vi "UserVars-Expand Repeat Value.vi"(7 "Expression":string) -> (8 "repeated values":dbl[](array[numeric]))   [LabVIEW 2020]
uses:
  <vilib>/regexp/Match Regular Expression.xnode
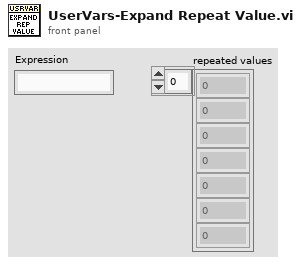
[diagram p1: front panel]
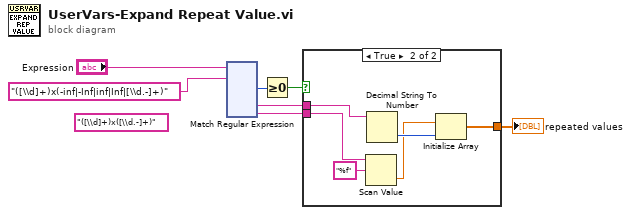
[diagram p0: block diagram]
diagram:
  (unwired) "([\\d]+)x([\\d.-]+)" ("regular expression")
  n1 = xnode "Match Regular Expression"("input string"="Expression", "regular expression"="([\\d]+)x(-inf|-Inf|inf|Inf|[\\d.-]+)") -> ("offset past match"=w6:i32, "submatch 1"=w5:string, "submatch 2"=w4:string)  [unwired: 4 in, 4 out]
  n2 = Greater Or Equal To 0?(x=w6) -> (x >= 0?=w2:bool)
  n3 = case shown="True" w2 {
    tunnel: w5 -> [_ w13]
    tunnel: w4 -> [_ w12]
    tunnel: [_ w8] -> w3
    frame False {
    }
    frame True {
      n4 = Scan Value(string=w12, format string="%f") -> (value=w9:dbl)  [unwired: 1 in, 1 out]
      n5 = Decimal String To Number(string=w13) -> (number=w10:i32)  [unwired: 2 in, 1 out]
      n6 = Initialize Array(w9, w10) -> (w8:dbl[])
    }
  }
  "repeated values" <- w3
